vi "SD Read Num Rarely.vi"(11 "Name":string="Numeric") -> (1 "Numeric":dbl)   [LabVIEW 2013]
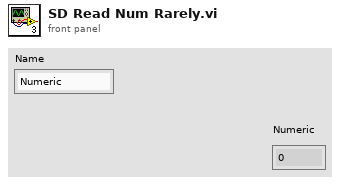
[diagram p1: front panel]
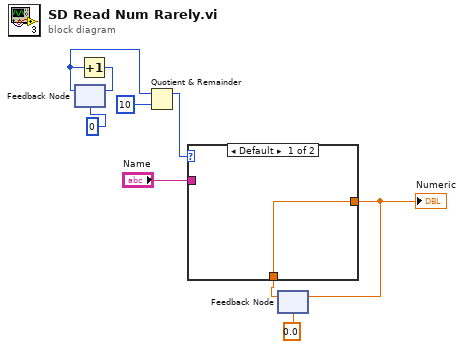
[diagram p0: block diagram]
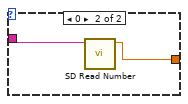
[diagram p2: hidden frame]
diagram:
  n1 = feedback #1(0) -> (w1:i32)
  n2 = Increment(x=w1) -> (x+1=w7:i32)
  n3 = feedback-in #1(w7) -> ()
  n4 = Quotient & Remainder(x=w1, y=10) -> (x-y*floor(x/y)=w5:i32)  [unwired: 1 out]
  n5 = feedback #2(0.0 ("Numeric")) -> (w3:dbl)
  n6 = case shown="Default" w5 {
    tunnel: "Name" -> [_ w12]
    tunnel: [w10 w11] -> w4
    tunnel: w3 -> [w10 _]
    frame Default {
    }
    frame 0 {
      n7 = call <vilib>:"SD Read Number.vi"("Name"=w12) -> ("Numeric"=w11:dbl)  [unwired: 8 in, 2 out]
    }
  }
  "Numeric" <- w4
  n8 = feedback-in #2(w4) -> ()
